vi "数据查询_校准记录.vi"() -> ()   [LabVIEW 2016]
uses:
  <vilib>/Utility/miscctls.llb/LVRowAndColumnUnsignedTypeDef.ctl
  <vilib>/Utility/miscctls.llb/LVPointTypeDef.ctl
  <userlib>/_OpenG.lib/array/array.llb/Sort 2D Array (String)__ogtk.vi
panel:
  out "确定查询":bool
  out "显示项":string[](array[string])
  out "condition":string
  in  "数据列表选择框":string(xcontrol)
  in  "导出":bool
  in  "条件筛选":bool
  in  "数据表":T1
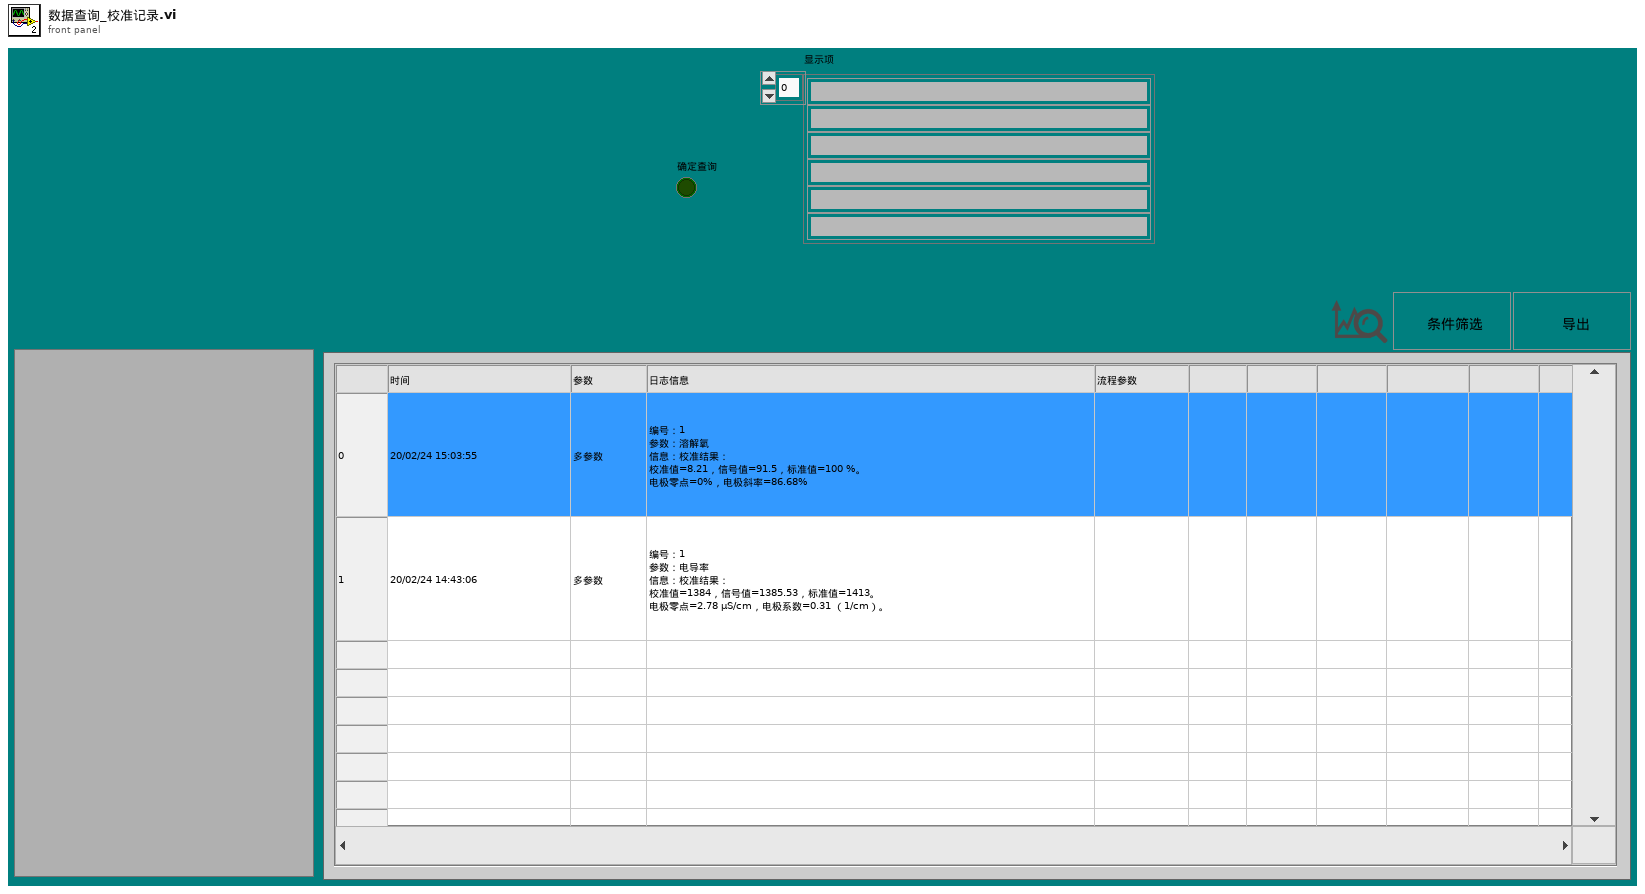
[diagram p1: front panel]
types:
  T1 = typedef "数据查询大列表框.ctl" = i32
  T2 = typedef "LVRowAndColumnUnsignedTypeDef.ctl" = cluster{"Row":u32, "Column":u32}
  T3 = typedef "LVPointTypeDef.ctl" = cluster{"Horizontal":i16, "Vertical":i16}
  T4 = enum8{"Enabled", "Disabled", "Disabled and Grayed Out"}
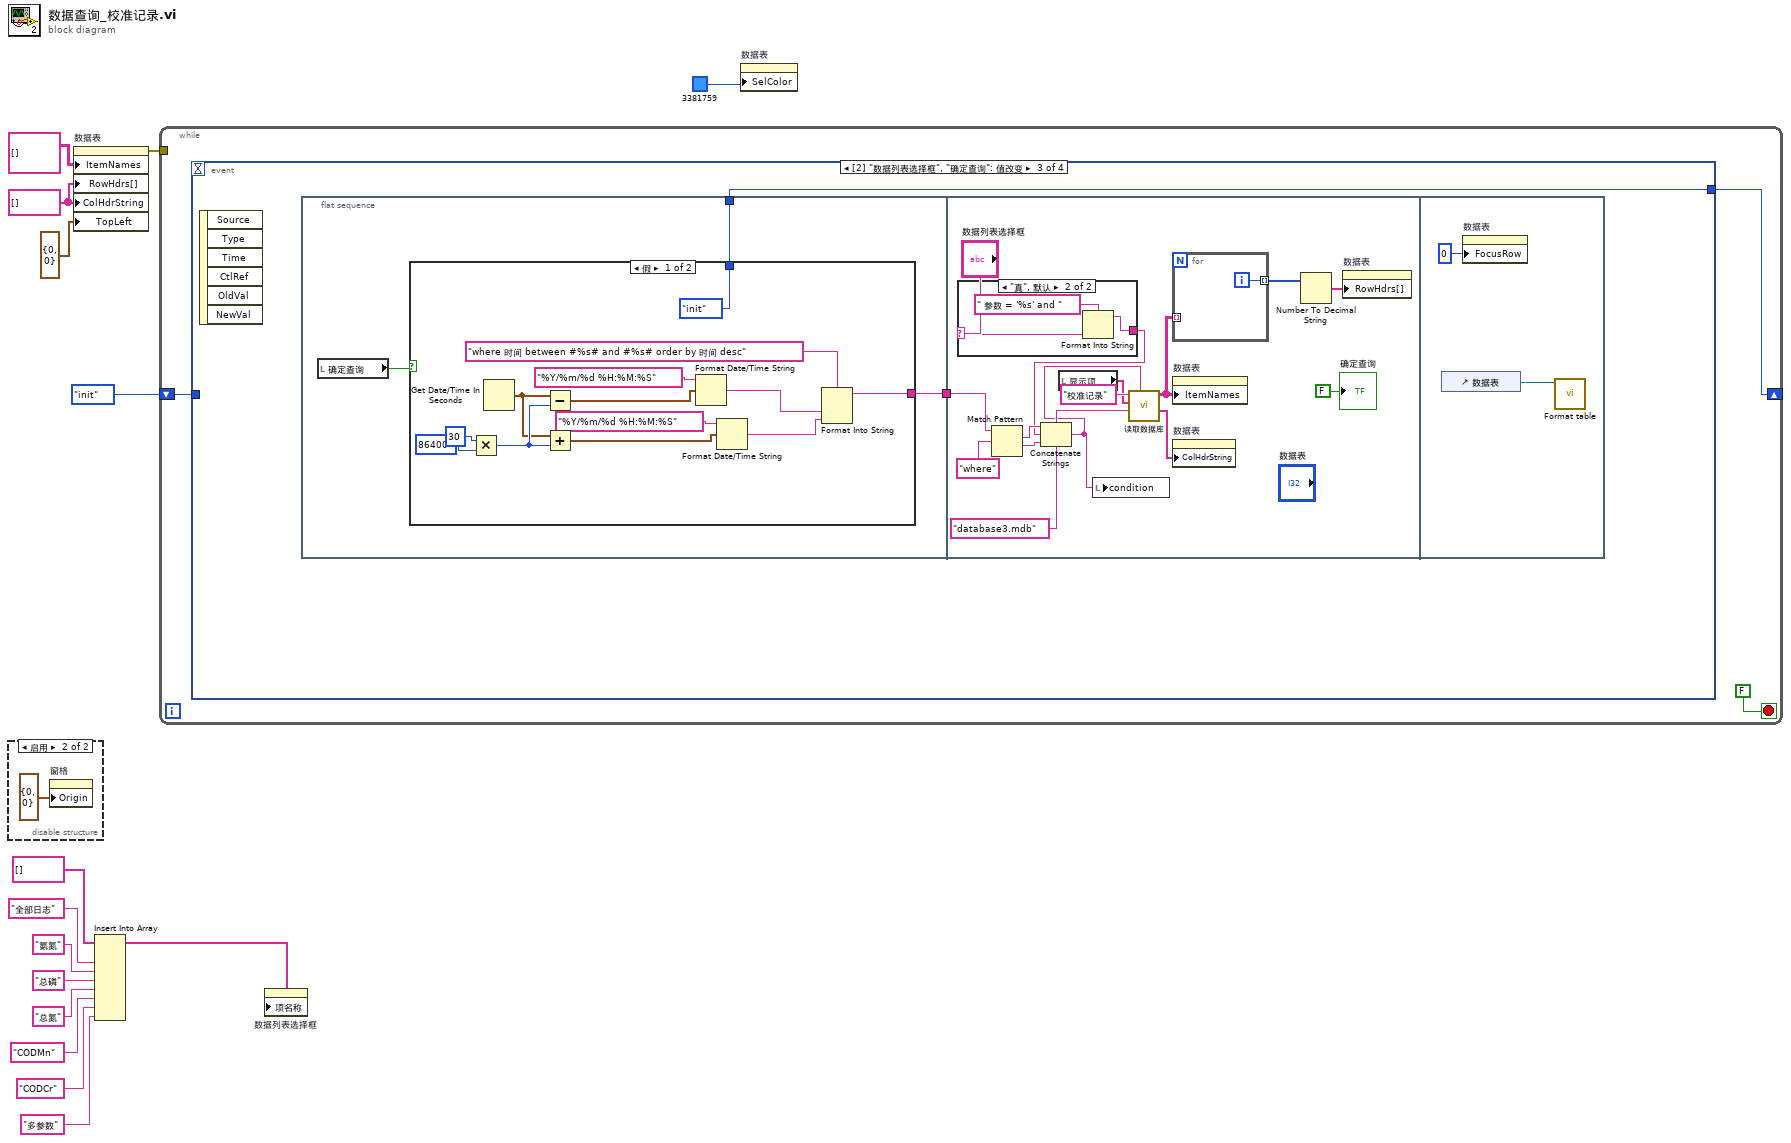
[diagram p0: block diagram]
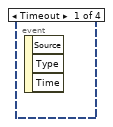
[diagram p2: hidden frame]
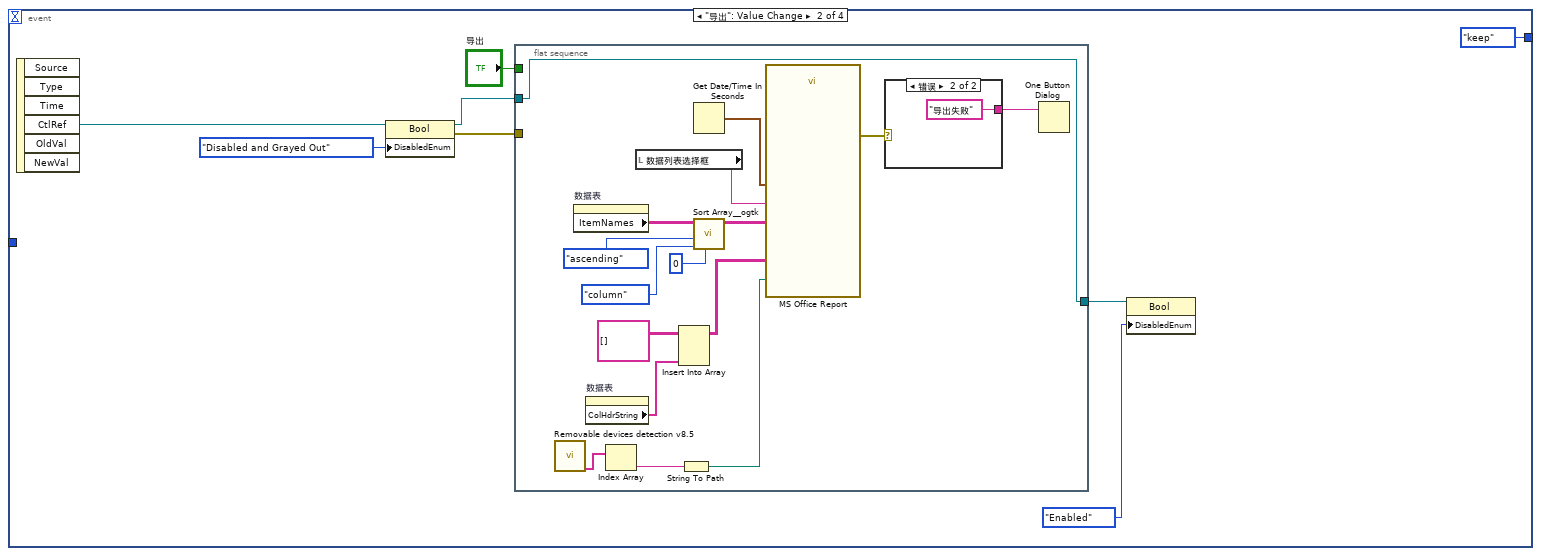
[diagram p3: hidden frame]
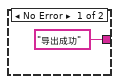
[diagram p4: hidden frame]
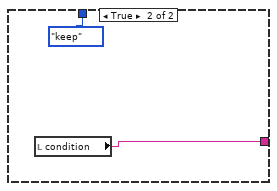
[diagram p5: hidden frame]
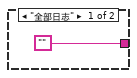
[diagram p6: hidden frame]
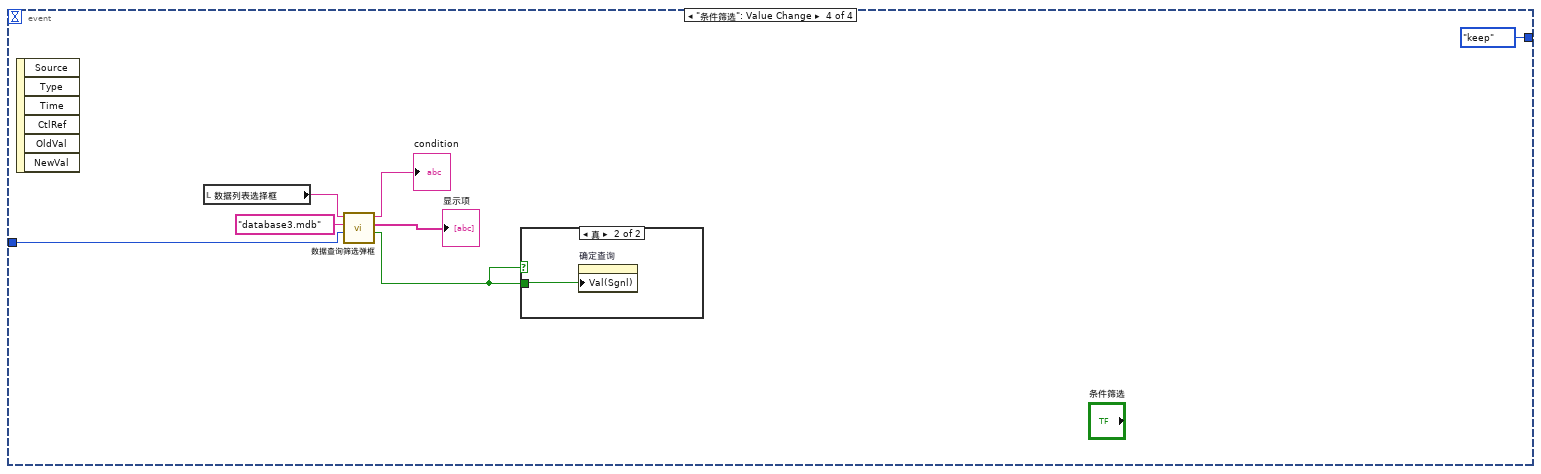
[diagram p7: hidden frame]
diagram:
  w5 = string[] [] ("行首字符串[]")
  n1 = disable-structure shown="启用" {
    frame Disabled {
    }
    frame Enabled {
      n2 = property on="窗格" class="Pane"("Origin"=T3 {"Horizontal"=0, "Vertical"=0} ("原点")) -> ()  [unwired: 2 in, 2 out]
    }
  }
  n3 = property on="数据表" class="MCListbox (严格)"("ItemNames"=string[][] [] ("项名"), "RowHdrs[]"=w5, "ColHdrString"=w5, "TopLeft"=T2 {"Row"=0, "Column"=0} ("左上可见单元格")) -> (error out=w7:errorcluster)  [unwired: 2 in, 1 out]
  n4 = Insert Into Array(array=string[] [], new element #1="全部日志" ("新元素/子数组"), new element #2="氨氮" ("新元素/子数组"), new element #3="总磷" ("新元素/子数组"), new element #4="总氮" ("新元素/子数组"), new element #5="CODMn" ("新元素/子数组"), new element #6="CODCr" ("新元素/子数组"), new element #7="多参数" ("新元素/子数组")) -> (w3:string[])  [unwired: 1 in]
  n5 = while {
    tunnel: w7 -> [_]
    shift-right: [w17] -> _
    shift-left: enum16{"init", "keep"}."init" ("是否初始化") -> [w18]
    stop <- FALSE stop-if-true
    n6 = event shown="[2] \"数据列表选择框\", \"确定查询\": 值改变" {
      selector: _ -> [_ _ _ _]
      dyn-events: _ -> [_ _ _ _]
      timeout: _ -> [_ _ _ _]
      tunnel: w18 -> [_ _ _ w89]
      tunnel: [_ enum16{"init", "keep"}."keep" ("是否初始化") w46 enum16{"init", "keep"}."keep" ("是否初始化")] -> w17
      event Timeout {
        n7 = event-data() -> ()  [unwired: 1 in, 3 out]
      }
      event "导出": Value Change {
        n8 = event-data() -> ("CtlRef"=w21:refnum<vi>)  [unwired: 1 in, 5 out]
        n9 = property class="Bool"(reference=w21, "DisabledEnum"=T4."Disabled and Grayed Out" ("禁用")) -> (reference out=w25:refnum<vi>, error out=w26:errorcluster)  [unwired: 1 in]
        n10 = flat-sequence {
          tunnel: w26 -> [_]
          tunnel: [w37] -> w24
          tunnel: w25 -> [w37]
          tunnel: "导出" -> [_]
          frame #0 {
            n11 = call "Removable devices detection v8.5.vi"() -> ("Removable"=w34:string[])  [unwired: 4 out]
            n12 = property on="数据表" class="MCListbox (严格)"() -> ("ItemNames"=w28:string[][])  [unwired: 2 in, 2 out]
            n13 = property on="数据表" class="MCListbox (严格)"() -> ("ColHdrString"=w30:string[])  [unwired: 2 in, 2 out]
            n14 = Index Array(array=w34) -> (element=w33:string)  [unwired: 1 in]
            n15 = local read "数据列表选择框"() -> (w38:string)
            n16 = Insert Into Array(array=string[][] [], new element=w30) -> (w29:string[][])  [unwired: 2 in]
            n17 = String To Path(string=w33) -> (path=w32:path)
            n18 = Get Date/Time In Seconds() -> (seconds since 1Jan1904=w43:timestamp)
            n19 = call-poly <userlib>:"Sort Array__ogtk.vi"("Column/Row to Sort By"=u32 0, "Sort By in"=enum16{"row", "column"}."column", "Order"=enum16{"ascending", "descending"}."ascending", "Array in"=w28) -> ("Sorted Array out"=w42:string[][])  [unwired: 4 in, 3 out]
            n20 = call "MS Office Report"("Path to Save Report"=w32, "导出日期"=w43, "监测参数"=w38, "数据输入"=w42, "字段定义"=w29) -> ("error out"=w36:errorcluster)  [unwired: 21 in, 1 out]
            n21 = case shown="错误" w36 {
              tunnel: ["导出成功" ("消息") "导出失败" ("消息")] -> w35
              frame No Error {
              }
              frame Error {
              }
            }
            n22 = One Button Dialog(message=w35) -> ()  [unwired: 1 in, 1 out]
          }
        }
        n23 = property class="Bool"(reference=w24, "DisabledEnum"=T4."Enabled" ("禁用")) -> ()  [unwired: 1 in, 2 out]
      }
      event "数据列表选择框", "确定查询": Value Change {
        n24 = event-data() -> ()  [unwired: 1 in, 6 out]
        n25 = flat-sequence {
          tunnel: [w49] -> w47
          tunnel: [w48] -> w46
          tunnel: w47 -> [w69]
          frame #0 {
            n26 = local read "确定查询"() -> (w50:bool)
            n27 = case shown="假" w50 {
              tunnel: [w52 w64] -> w49
              tunnel: [enum16{"init", "keep"}."init" ("是否初始化") enum16{"init", "keep"}."keep" ("是否初始化")] -> w48
              frame False {
                n28 = Multiply(x=30, y=86400) -> (x*y=w54:i32)
                n29 = Get Date/Time In Seconds() -> (seconds since 1Jan1904=w53:timestamp)
                n30 = Subtract(x=w53, y=w54) -> (x-y=w60:timestamp)
                n31 = Add(x=w53, y=w54) -> (x+y=w59:timestamp)
                n32 = Format Date/Time String(time format string (%c)="%Y/%m/%d %H:%M:%S" ("时间格式字符串(%c)"), seconds (now)=w60) -> (date/time string=w62:string)  [unwired: 1 in]
                n33 = Format Date/Time String(time format string (%c)="%Y/%m/%d %H:%M:%S" ("时间格式字符串(%c)"), seconds (now)=w59) -> (date/time string=w63:string)  [unwired: 1 in]
                n34 = Format Into String(format string="where 时间 between #%s# and #%s# order by 时间 desc", w62, w63) -> (resulting string=w52:string)  [unwired: 2 in, 1 out]
              }
              frame True {
                n35 = local read "condition"() -> (w64:string)
              }
            }
          }
          frame #1 {
            n36 = case shown="\"真\", 默认" "数据列表选择框" {
              selector: "数据列表选择框" -> [_ w83]
              tunnel: ["" w82] -> w70
              frame "全部日志" {
              }
              frame "真", Default {
                n37 = Format Into String(format string=" 参数 = '%s' and " ("condition"), w83) -> (resulting string=w82:string)  [unwired: 2 in, 1 out]
              }
            }
            n38 = Match Pattern(string=w69, regular expression="where") -> (match substring=w72:string, after substring=w71:string)  [unwired: 1 in, 2 out]
            n39 = Concatenate Strings(w72, w70, w71) -> (w67:string)
            n40 = local read "显示项"() -> (w68:string[])
            n41 = local write "condition"(w67) -> ()
            n42 = call "读取数据库.vi"("condition"=w67, "database"="database3.mdb", "显示项"=w68, "组合框"="校准记录" ("字符串")) -> ("columns"=w80:string[], "表格"=w75:string[][])  [unwired: 4 in, 2 out]
            n43 = for {
              tunnel: w75 -> [_] mode=indexing
              tunnel: [w85] -> w79 mode=indexing
              i -> [w85]
            }
            n44 = property on="数据表" class="MCListbox (严格)"("ItemNames"=w75) -> ()  [unwired: 2 in, 2 out]
            n45 = property on="数据表" class="MCListbox (严格)"("ColHdrString"=w80) -> ()  [unwired: 2 in, 2 out]
            n46 = Number To Decimal String(number=w79) -> (decimal integer string=w78:string[])  [unwired: 1 in]
            n47 = property on="数据表" class="MCListbox (严格)"("RowHdrs[]"=w78) -> ()  [unwired: 2 in, 2 out]
            "确定查询" <- FALSE ("确定查询")
          }
          frame #2 {
            n48 = control-ref of="数据表"() -> (w86:refnum<vi>)
            n49 = property on="数据表" class="MCListbox (严格)"("FocusRow"=0 ("选中行")) -> ()  [unwired: 2 in, 2 out]
            n50 = call "Format table.vi"("Table输入"=w86) -> ()  [unwired: 11 in]
          }
        }
      }
      event "条件筛选": Value Change {
        n51 = event-data() -> ()  [unwired: 1 in, 6 out]
        n52 = local read "数据列表选择框"() -> (w90:string)
        n53 = call "数据查询筛选弹框.vi"("是否初始化"=w89, "database"="database3.mdb", "table"=w90) -> ("确定输出"=w92:bool, "显示项"=→"显示项":string[], "condition"=→"condition":string)  [unwired: 5 in, 1 out]
        n54 = case shown="真" w92 {
          tunnel: w92 -> [_ w95]
          frame False {
          }
          frame True {
            n55 = property on="确定查询" class="Bool (严格)"("Val(Sgnl)"=w95) -> ()  [unwired: 2 in, 2 out]
          }
        }
      }
    }
  }
  n56 = property on="数据列表选择框" class="数据列表选择框 (严格)"("项名称"=w3) -> ()  [unwired: 2 in, 2 out]
  n57 = property on="数据表" class="MCListbox (严格)"("SelColor"=u32 3381759) -> ()  [unwired: 2 in, 2 out]
